vi "get_TIFF_page_properties.vi"(8 "error in (no error)":errorcluster, 10 "page":i32, 11 "path in":path) -> (0 "error out":errorcluster, 1 "height":i32, 2 "width":i32, 3 "path out":path, 4 "number of bytes":i32, 5 "bits per sample":i32, 7 "samples per pixel":i32)   [LabVIEW 2010, in "TIFFManagement.lvlib"]
uses:
  TIFFManagement.lvlib
  VisualCPP/Release/TIFFManagement.dll
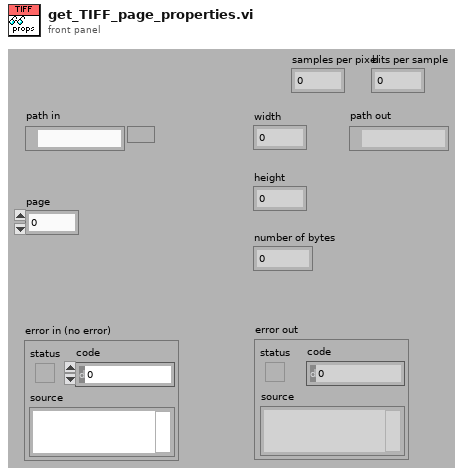
[diagram p1: front panel]
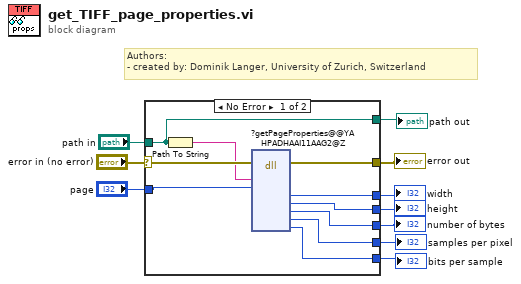
[diagram p0: block diagram]
diagram:
  # "Authors: \n- created by: Dominik Langer, University of Zurich, Switzerland"
  n1 = case shown="No Error" "error in (no error)" {
    selector: "error in (no error)" -> [w20 w22]
    tunnel: "path in" -> [w13 w21]
    tunnel: "page" -> [w17 _]
    tunnel: [w19 w22] -> w7
    tunnel: [w16 _] -> w6
    tunnel: [w15 _] -> w5
    tunnel: [w14 _] -> w4
    tunnel: [w13 w21] -> w3
    tunnel: [w12 _] -> w2
    tunnel: [w11 _] -> w1
    frame No Error {
      n2 = Path To String(path=w13) -> (string=w18:string)
      n3 = dll-call lib="C:/helioscan/common/libraries/TIFFManagement/VisualCPP/Release/TIFFManagement.dll" fn="?getPageProperties@@YAHPADHAAI11AAG2@Z" label="getPageSize()"(error in=w20, "path"=w18, "page"=w17) -> (error out=w19:errorcluster, "width"=w16:i32, "height"=w15:i32, "number of bytes"=w14:i32, "samplesPerPixel"=w12:i32, "bitsPerSample"=w11:i32)  [unwired: 10 in, 1 out]
    }
    frame Error {
    }
  }
  "error out" <- w7
  "width" <- w6
  "height" <- w5
  "number of bytes" <- w4
  "path out" <- w3
  "samples per pixel" <- w2
  "bits per sample" <- w1
